vi "Simulation Input Global.vi"() -> ()   [LabVIEW 2017]
panel:
  out "Top SW":bool
  out "Bottom SW":bool
  in  "BottomDist":dbl
  in  "Sim Gripper Input R":dbl
  in  "Sim Gripper Input L":dbl
  in  "Sim Elevator Input":dbl
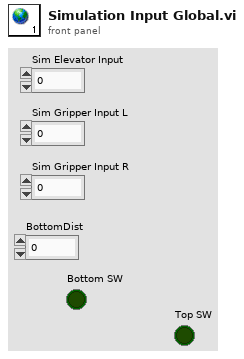
[diagram p1: front panel]
diagram:
